vi "CalcMatrix.vi"(8 "error in (no error)":errorcluster, 11 "MultiBandState in":refnum<class "MultiBandState.lvclass">) -> (0 "error out":errorcluster, 3 "MultiBandState out":refnum<class "MultiBandState.lvclass">)   [LabVIEW 2014, in "Functions.lvlib" / "MultiBandState.lvclass"]
uses:
  MultiBandState.lvclass
  <vilib>/Analysis/Matrix/Datatypes/RealMatrix.ctl
  MultiBandState.lvclass/MultiBandState.ctl
  <vilib>/Analysis/7linalg.llb/Real Matrix Exp.vi
  Accessors/Read MultiBand.vi
  Accessors/Read SampleRate.vi
  Accessors/Write MultiBand.vi
  <vilib>/Utility/error.llb/Error Cluster From Error Code.vi
  <vilib>/Analysis/Matrix/Numeric/Multiply/Multiply - R,RM.vi
  <vilib>/ErrorRing/Error Ring.xnode
  <vilib>/Analysis/Matrix/NI_Matrix.lvlib
  <vilib>/Analysis/NI_AALBase.lvlib
panel:
  out "Real Matrix":T1
  in  "Channels":T2(array[cluster])
  # "Band"
  # "Band"
  # "Band"
  # "Band"
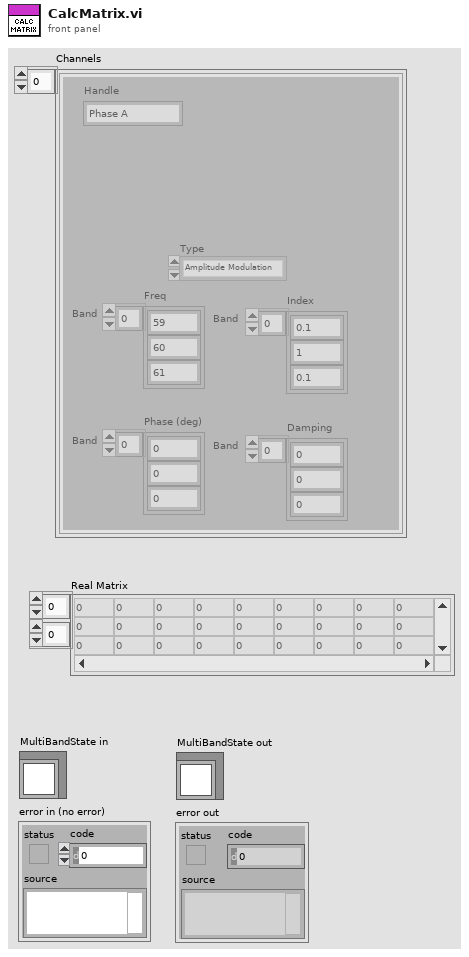
[diagram p1: front panel]
types:
  T1 = typedef "NI_Matrix.lvlib/RealMatrix.ctl" = dbl[][]
  T2 = cluster{"Freq":dbl[], "Index":dbl[], "Phase (deg)":dbl[], "Type":enum16{"Multiband", "Amplitude Modulation", "Phase Modulation"}, "Damping":dbl[], "Handle":string}[]
  T3 = cluster{"Handle":string, "Size":i32, "Gain":dbl, "Offset":dbl, "A":T1, "B":T1, "C":T1, "D":T1, "X":T1, "Waveform":waveform(dbl)}[]
  T4 = cluster{"Handle":string, "Size":i32, "Gain":dbl, "Offset":dbl, "A":T1, "B":T1, "C":T1, "D":T1, "X":T1, "Waveform":waveform(dbl)}
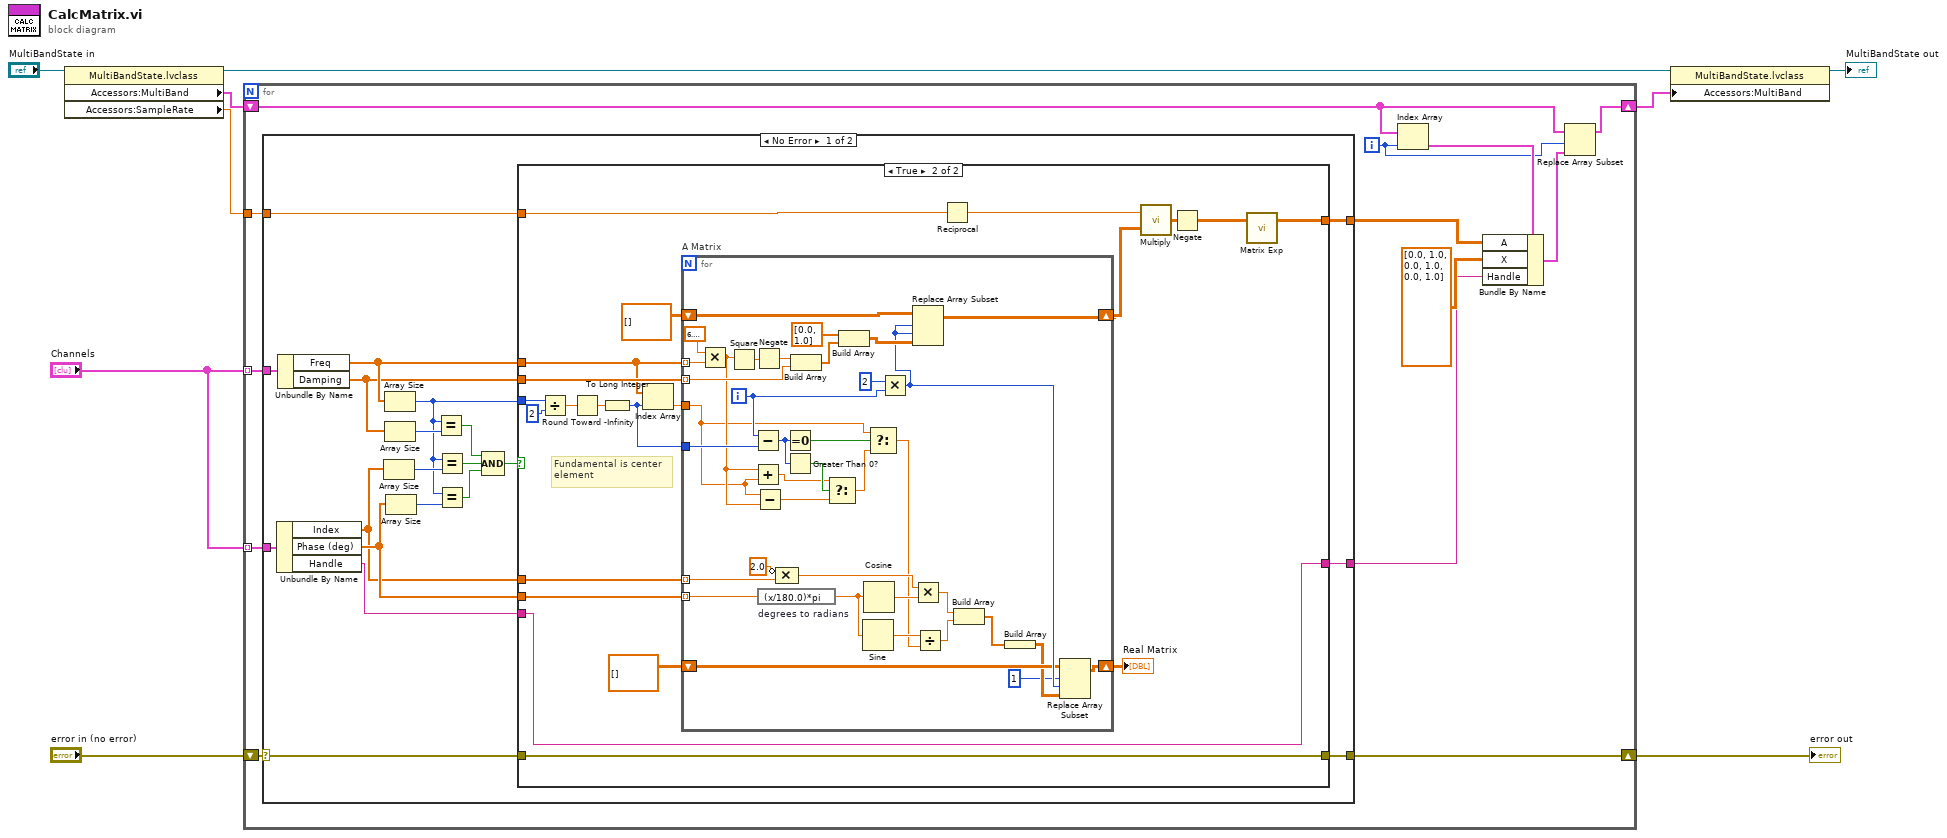
[diagram p0: block diagram]
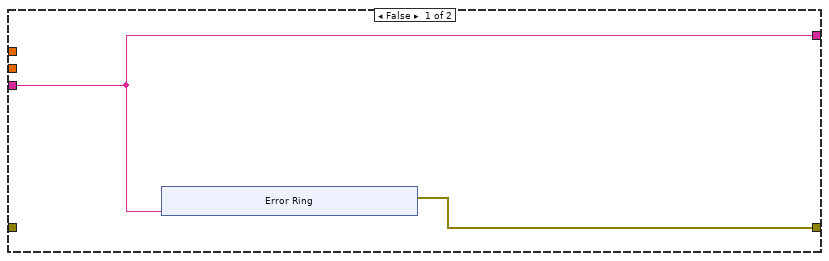
[diagram p2: hidden frame]
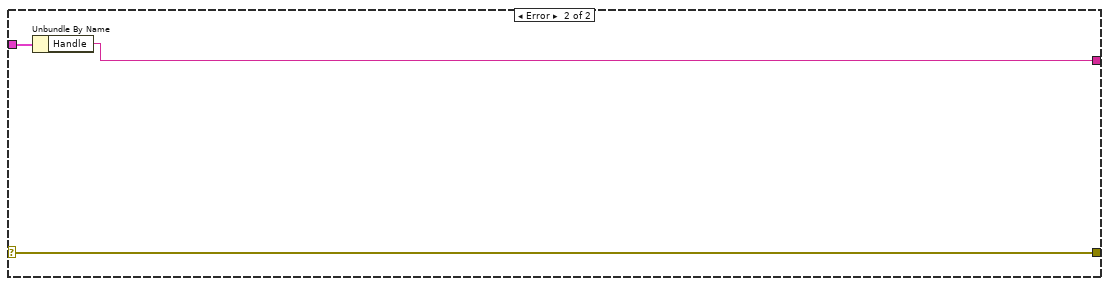
[diagram p3: hidden frame]
diagram:
  n1 = property class="MultiBandState.lvclass"(reference="MultiBandState in") -> (reference out=w5:refnum<class "MultiBandState.lvclass">, "Accessors:MultiBand"=w4:T3, "Accessors:SampleRate"=w1:dbl)  [unwired: 1 in, 1 out]
  n2 = for {
    tunnel: "Channels" -> [w22] mode=indexing
    tunnel: "Channels" -> [w21] mode=indexing
    shift-right: [w19] -> w8
    shift-left: "error in (no error)" -> [w20]
    shift-right: [w13] -> w2
    shift-left: w4 -> [w14]
    tunnel: w1 -> [w10]
    i -> [w16]
    n3 = case shown="No Error" w20 {
      selector: w20 -> [w31 w112]
      tunnel: w22 -> [w42 _]
      tunnel: w21 -> [w38 w111]
      tunnel: [w30 w112] -> w19
      tunnel: [w27 _] -> w17
      tunnel: [w26 w110] -> w11
      tunnel: w10 -> [w25 _]
      frame No Error {
        n4 = Unbundle By Name(w38) -> ("Index"=w28:dbl[], "Phase (deg)"=w29:dbl[], "Handle"=w24:string)
        n5 = Unbundle By Name(w42) -> ("Freq"=w41:dbl[], "Damping"=w40:dbl[])
        n6 = Array Size(array=w28) -> (size(s)=w37:i32)
        n7 = Array Size(array=w41) -> (size(s)=w23:i32)
        n8 = Array Size(array=w40) -> (size(s)=w39:i32)
        n9 = Array Size(array=w29) -> (size(s)=w36:i32)
        n10 = Equal?(x=w23, y=w39) -> (x = y?=w35:bool)
        n11 = Equal?(x=w23, y=w37) -> (x = y?=w34:bool)
        n12 = Equal?(x=w23, y=w36) -> (x = y?=w33:bool)
        n13 = Compound Arithmetic op=AND(w35, w34, w33) -> (w32:bool)
        n14 = case shown="True" w32 {
          tunnel: w41 -> [_ w56]
          tunnel: w40 -> [_ w71]
          tunnel: w31 -> [_ w70]
          tunnel: [w44 w70] -> w30
          tunnel: w29 -> [_ w62]
          tunnel: w28 -> [_ w63]
          tunnel: [_ w68] -> w27
          tunnel: [w43 w61] -> w26
          tunnel: w25 -> [_ w69]
          tunnel: w24 -> [w43 w61]
          tunnel: w23 -> [_ w60]
          frame False {
            n15 = xnode "Error Ring"("parameter 0"=w43) -> ("error out"=w44:errorcluster)
          }
          frame True {
            # "Fundamental is center\nelement"
            n16 = Divide(x=w60, y=2) -> (x/y=w58:dbl)
            n17 = Round Toward -Infinity(1:w58) -> (0:w57:dbl)
            n18 = To Long Integer(number=w57) -> (32bit integer=w54:i32)
            n19 = Index Array(array=w56, index=w54) -> (element=w55:dbl)
            n20 = for "A Matrix" {
              shift-right: [w109] -> w67
              shift-left: T1 [] ("Real Matrix") -> [w108]
              tunnel: w56 -> [w101] mode=indexing
              tunnel: w71 -> [w105] mode=indexing
              tunnel: w63 -> [w99] mode=indexing
              tunnel: w62 -> [w97] mode=indexing
              tunnel: w55 -> [w87]
              tunnel: w54 -> [w92]
              shift-right: [w76] -> w52
              shift-left: T1 [] ("Real Matrix") -> [w77]
              i -> [w91]
              n21 = Multiply(x=6.283185307179586, y=w101) -> (x*y=w88:dbl)
              n22 = Square(x=w88) -> (x^2=w107:dbl)
              n23 = Subtract(x=w91, y=w92) -> (x-y=w89:i32)
              n24 = Add(x=w88, y=w87) -> (x+y=w85:dbl)
              n25 = Negate(x=w107) -> (-x=w106:dbl)
              n26 = Subtract(x=w87, y=w88) -> (x-y=w84:dbl)
              n27 = expression code="(x/180.0)*pi" "degrees to radians"(w97) -> (w96:dbl)
              n28 = Compound Arithmetic op=MULTIPLY(invert 2.0 ("value"), w99) -> (w94:dbl)
              n29 = Equal To 0?(x=w89) -> (x = 0?=w90:bool)
              n30 = Greater Than 0?(x=w89) -> (x > 0?=w86:bool)
              n31 = Build Array(w106, w105) -> (w103:dbl[])
              n32 = Select(t=w85, s=w86, f=w84) -> (s? t:f=w83:dbl)
              n33 = Build Array(dbl[] [0.0, 1.0], w103) -> (w102:dbl[][])
              n34 = Sine(x=w96) -> (sin(x)=w82:dbl)
              n35 = Cosine(x=w96) -> (cos(x)=w95:dbl)
              n36 = Select(t=w87, s=w90, f=w83) -> (s? t:f=w81:dbl)
              n37 = Multiply(x=2 ("y"), y=w91) -> (x*y=w78:i32)
              n38 = Replace Array Subset(array=w108, new element=w102, index (row)=w78, index (col)=w78) -> (w109:T1)
              n39 = Multiply(x=w94, y=w95) -> (x*y=w80:dbl)
              n40 = Divide(x=w82, y=w81) -> (x/y=w79:dbl)
              n41 = Build Array(w80, w79) -> (w75:dbl[])
              n42 = Build Array(w75) -> (w74:dbl[][])
              n43 = Replace Array Subset(array=w77, new element=w74, index (row)=1 ("disabled index (row)"), index (col)=w78) -> (w76:T1)
            }
            "Real Matrix" <- w52
            n44 = Reciprocal(x=w69) -> (1/x=w66:dbl)
            n45 = call-poly <vilib>:"Multiply.vi"("Real Matrix A"=w67, "Real Scalar c"=w66) -> ("c * A"=w65:T1)
            n46 = Negate(x=w65) -> (-x=w64:T1)
            n47 = call-poly <vilib>:"Matrix Exp.vi"("Input Matrix"=w64) -> ("Matrix Exp"=w68:T1)  [unwired: 1 in, 1 out]
          }
        }
      }
      frame Error {
        n48 = Unbundle By Name(w111) -> ("Handle"=w110:string)
      }
    }
    n49 = Index Array(array=w14, index=w16) -> (element=w18:T4)
    n50 = Bundle By Name(cluster=w18, "A"=w17, "X"=T1 [[0.0], [1.0], [0.0], [1.0], [0.0], [1.0]], "Handle"=w11) -> (w15:T4)
    n51 = Replace Array Subset(array=w14, new element=w15, index=w16) -> (w13:T3)
  }
  "error out" <- w8
  n52 = property class="MultiBandState.lvclass"(reference=w5, "Accessors:MultiBand"=w2) -> (reference out=→"MultiBandState out":refnum<class "MultiBandState.lvclass">)  [unwired: 1 in, 1 out]
